vi "PNA_SWEEP MODE.vi"(4 "Mode":i32(ring) items=["HOLD", "CONT", "GROUP", "SINGLE"], 6 "Channel":i32=1, 8 "error in (no error)":errorcluster, 11 "VISA resource name":refnum<visa-resource-name>) -> (0 "error out":errorcluster, 3 "VISA resource name out":refnum<visa-resource-name>)   [LabVIEW 2018, in "Agilent ENA Series.lvlib"]
doc: "Changes the state of each channel of selected channel to the startup state in the trigger system.\n\nWhen this function is executed for a channel in the idle state, it goes into the initiate state immediately. Then, after measurement is executed once, it goes back to the idle state.\n\nIf this function is executed for a channel that is not in the idle state or for which the continuous initiation mode is enabled, an error occurs."
uses:
  Agilent ENA Series.lvlib
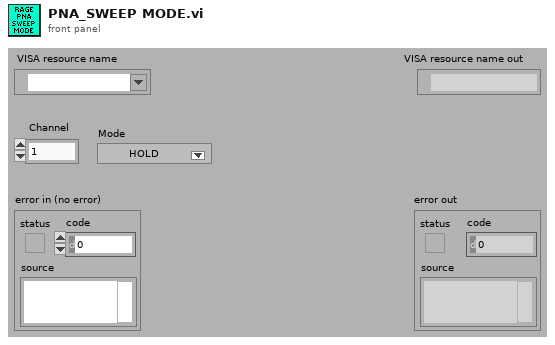
[diagram p1: front panel]
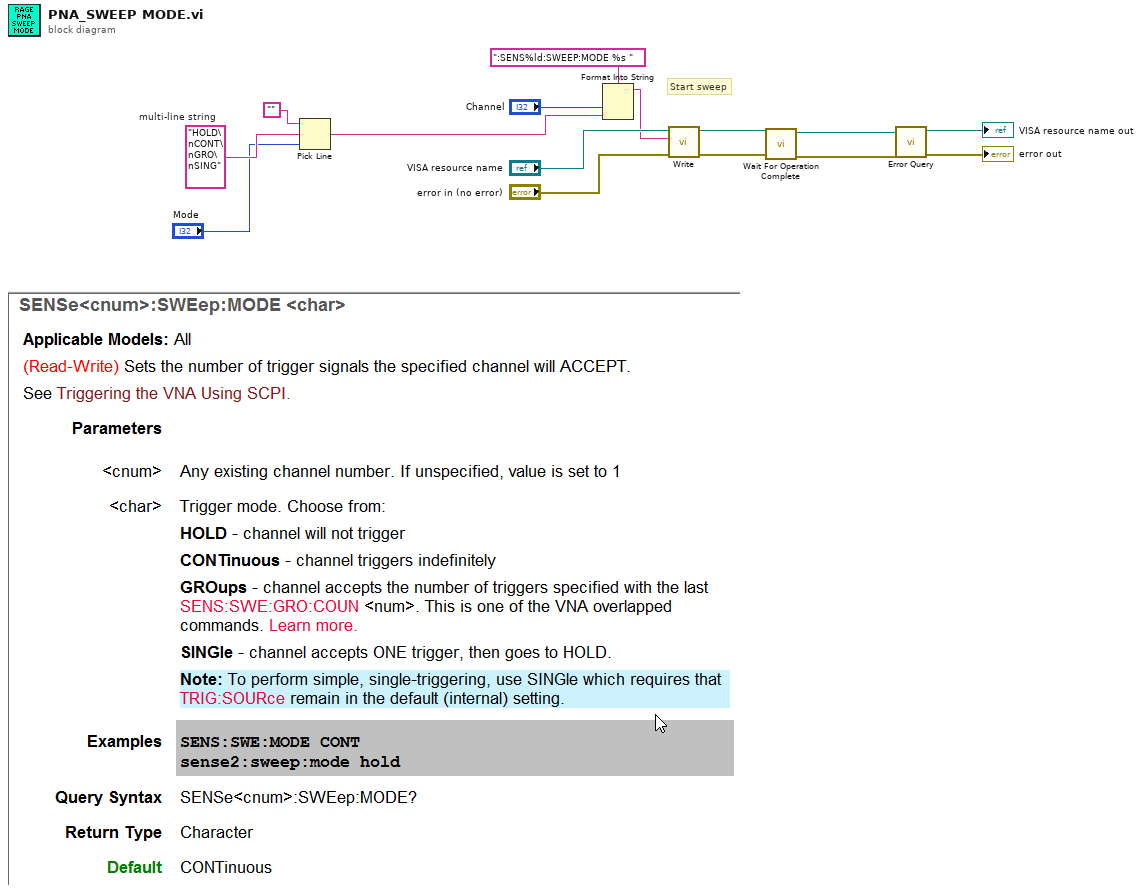
[diagram p0: block diagram]
diagram:
  w8 = "HOLD\nCONT\nGRO\nSING"  # multi-line string
  # "Start sweep"
  n1 = Pick Line(string ("")="", multi-line string=w8, line index="Mode") -> (output string=w6:string)
  n2 = Format Into String(format string=":SENS%ld:SWEEP:MODE %s ", "Channel", w6) -> (resulting string=w11:string)  [unwired: 2 in, 1 out]
  n3 = call "Write.vi"("error in (no error)"="error in (no error)", "String ()"=w11, "VISA resource name"="VISA resource name") -> ("error out"=w4:errorcluster, "VISA resource name out"=w3:refnum<visa-resource-name>)  [unwired: 6 in, 1 out]
  n4 = call "Wait For Operation Complete.vi"("error in (no error)"=w4, "VISA resource name"=w3) -> ("error out"=w1:errorcluster, "VISA resource name out"=w2:refnum<visa-resource-name>)  [unwired: 8 in]
  n5 = call "Error Query.vi"("error in (no error)"=w1, "VISA resource name"=w2) -> ("error out"=→"error out":errorcluster, "VISA resource name out"=→"VISA resource name out":refnum<visa-resource-name>)  [unwired: 6 in, 2 out]
